vi "字符串与实际变量转换-配置和标定参数.vi"(4 "配置和标定参数":string[](array[string])) -> ()   [LabVIEW 2013]
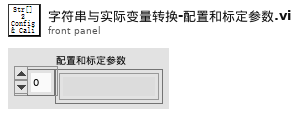
[diagram p1: front panel]
types:
  T1 = cluster{"卡件工作模式":enum32{"未接入", "直流型", "交流型", "交流型 2"}, "转速反馈":enum32{"未接入", "直流型"}, "故障输出模式":enum32{"未接入", "直流型", "交流型"}, "DEH类型":enum32{"内置", "外接"}, "LVDT 2类型":enum32{"未接入", "直流", "交流"}, "LVDT 1类型":enum32{"未接入", "直流", "交流"}, "阀门电流输出量程":enum32{"-200~200 mA", "-50~50 mA", "-27~27 mA", "4~20 mA", "0~200 mA"}, "DEH内置参数值":dbl, "测速盘齿数":u32, "最高转速":u32, "最低转速":u32, "速差曲线点1 反馈":dbl, "速差曲线点3 反馈":dbl, "速差曲线点2 反馈":dbl, "速差曲线点4 反馈":dbl, "速差曲线点1":dbl, "速差曲线点3":dbl, "速差曲线点2":dbl, "速差曲线点4":dbl, "比例调节增益":dbl, "积分调节时间":dbl, "DEH零度标定":i32, "DEH满度标定":i32, "LVDT 2零度标定":i32, "LVDT 2满度标定":i32, "LVDT 1零度标定":i32, "LVDT 1满度标定":i32, "输出电流上限值":u32, "输出电流零值":u32, "输出电流下限值":u32, "表头20mA输出值":u16, "表头4mA输出值":u16, "反向偏差":dbl, "正向偏差":dbl, "自动标定延时时间":dbl, "转速零度标定":i16, "转速满度标定":i16, "转速指令采样值":i16, "标准最高转速":dbl, "标准最低转速":dbl}
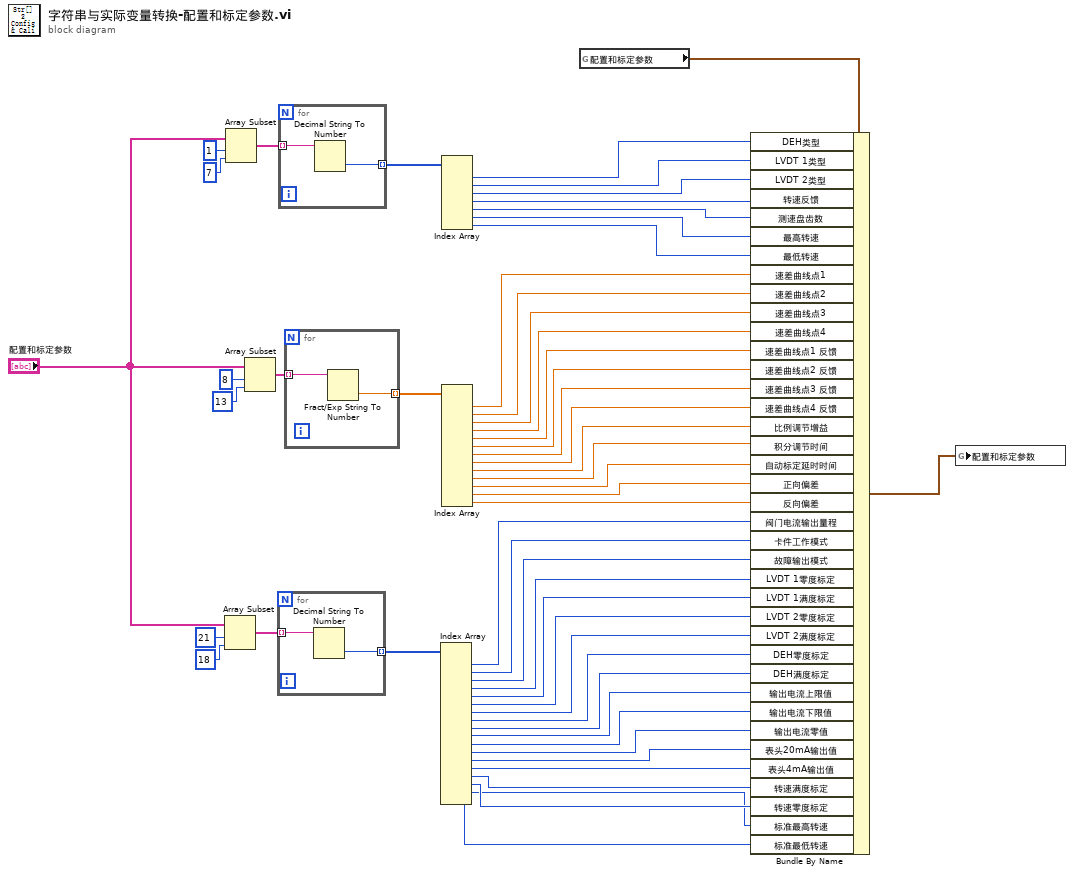
[diagram p0: block diagram]
diagram:
  n1 = Array Subset(array="配置和标定参数", index=21, length=18) -> (w21:string[])
  n2 = Array Subset(array="配置和标定参数", index=1, length=7) -> (w45:string[])
  n3 = Array Subset(array="配置和标定参数", index=8, length=13) -> (w51:string[])
  n4 = for {
    tunnel: w21 -> [w55] mode=indexing
    tunnel: [w54] -> w20 mode=indexing
    n5 = Decimal String To Number(string=w55) -> (number=w54:i32)  [unwired: 2 in, 1 out]
  }
  n6 = for {
    tunnel: w45 -> [w57] mode=indexing
    tunnel: [w56] -> w44 mode=indexing
    n7 = Decimal String To Number(string=w57) -> (number=w56:i32)  [unwired: 2 in, 1 out]
  }
  n8 = for {
    tunnel: w51 -> [w59] mode=indexing
    tunnel: [w58] -> w50 mode=indexing
    n9 = Fract/Exp String To Number(string=w59) -> (number=w58:dbl)  [unwired: 3 in, 1 out]
  }
  n10 = Index Array(array=w20) -> (element #1=w18:i32, element #2=w17:i32, element #3=w16:i32, element #4=w15:i32, element #5=w14:i32, element #6=w13:i32, element #7=w12:i32, element #8=w11:i32, element #9=w10:i32, element #10=w9:i32, element #11=w8:i32, element #12=w7:i32, element #13=w6:i32, element #14=w5:i32, element #15=w4:i32, element #16=w3:i32, element #17=w2:i32, element #18=w1:i32)  [unwired: 18 in]
  n11 = Index Array(array=w44) -> (element #1=w43:i32, element #2=w42:i32, element #3=w41:i32, element #4=w40:i32, element #5=w39:i32, element #6=w38:i32, element #7=w37:i32)  [unwired: 7 in]
  n12 = Index Array(array=w50) -> (element #1=w36:dbl, element #2=w35:dbl, element #3=w34:dbl, element #4=w33:dbl, element #5=w32:dbl, element #6=w31:dbl, element #7=w30:dbl, element #8=w29:dbl, element #9=w28:dbl, element #10=w27:dbl, element #11=w26:dbl, element #12=w25:dbl, element #13=w24:dbl)  [unwired: 13 in]
  n13 = global read "配置和标定参数.vi" "配置和标定参数"() -> (w49:T1)
  n14 = Bundle By Name(cluster=w49, "DEH类型"=w43, "LVDT 1类型"=w42, "LVDT 2类型"=w41, "转速反馈"=w40, "测速盘齿数"=w39, "最高转速"=w38, "最低转速"=w37, "速差曲线点1"=w36, "速差曲线点2"=w35, "速差曲线点3"=w34, "速差曲线点4"=w33, "速差曲线点1 反馈"=w32, "速差曲线点2 反馈"=w31, "速差曲线点3 反馈"=w30, "速差曲线点4 反馈"=w29, "比例调节增益"=w28, "积分调节时间"=w27, "自动标定延时时间"=w26, "正向偏差"=w25, "反向偏差"=w24, "阀门电流输出量程"=w18, "卡件工作模式"=w17, "故障输出模式"=w16, "LVDT 1零度标定"=w15, "LVDT 1满度标定"=w14, "LVDT 2零度标定"=w13, "LVDT 2满度标定"=w12, "DEH零度标定"=w11, "DEH满度标定"=w10, "输出电流上限值"=w9, "输出电流下限值"=w8, "输出电流零值"=w7, "表头20mA输出值"=w6, "表头4mA输出值"=w5, "转速满度标定"=w4, "转速零度标定"=w3, "标准最高转速"=w2, "标准最低转速"=w1) -> (w48:T1)
  n15 = global write "配置和标定参数.vi" "配置和标定参数"(w48) -> ()
